vi "Check Value.vi"(6 "Coerce Value? (F)":bool, 7 "Column Configuration":refnum<class "Column Configuration.lvclass">, 8 "error in (no error)":errorcluster, 9 "Value Type":refnum<class "Value Type.lvclass">, 10 "Value In":variant, 11 "Check Manager in":refnum<class "Constraint Manager.lvclass">) -> (0 "error out":errorcluster, 2 "Value Out":variant, 3 "Check Manager out":refnum<class "Constraint Manager.lvclass">)   [LabVIEW 2020, in "Composed Columns.lvlib" / "Constraint Manager.lvclass"]
uses:
  Constraint Manager.lvclass
  Value Type/Value Type.lvclass
  Basic Columns/Column Configuration/Basic Column Configuration Class/Column Configuration.lvclass
  Constraint Manager.lvclass/Constraint Manager.ctl
  Check/Constraint.lvclass
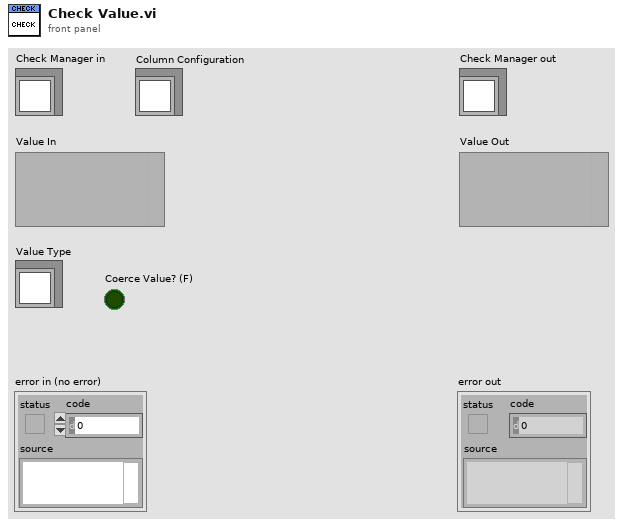
[diagram p1: front panel]
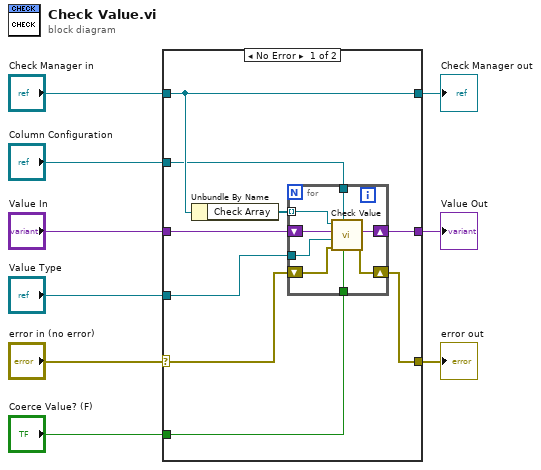
[diagram p0: block diagram]
diagram:
  n1 = case shown="No Error" "error in (no error)" {
    selector: "error in (no error)" -> [w12 w28]
    tunnel: "Check Manager in" -> [w18 w29]
    tunnel: [w18 w29] -> w7
    tunnel: [w11 w28] -> w6
    tunnel: "Coerce Value? (F)" -> [w16 _]
    tunnel: "Value In" -> [w15 w27]
    tunnel: "Column Configuration" -> [w14 _]
    tunnel: "Value Type" -> [w13 _]
    tunnel: [w10 w27] -> w1
    frame No Error {
      n2 = Unbundle By Name(w18) -> ("Check Array"=w17:refnum<class "Constraint.lvclass">[])
      n3 = for {
        tunnel: w17 -> [w26] mode=indexing
        tunnel: w16 -> [w25]
        shift-right: [w23] -> w10
        shift-left: w15 -> [w24]
        tunnel: w14 -> [w22]
        tunnel: w13 -> [w21]
        shift-right: [w19] -> w11
        shift-left: w12 -> [w20]
        n4 = call-dynamic "Check Value.vi"("Coerce Value? (F)"=w25, "Column Configuration"=w22, "error in (no error)"=w20, "Value Type"=w21, "Value In"=w24, "Check in"=w26) -> ("error out"=w19:errorcluster, "Value Out"=w23:variant)  [unwired: 3 in, 1 out]
      }
    }
    frame Error {
    }
  }
  "error out" <- w6
  "Check Manager out" <- w7
  "Value Out" <- w1
